vi "Draw_polygon_exercise_ms.vi"() -> ()   [LabVIEW 2016]
uses:
  Classes/Controller/Motion/A3200 Folder/A3200.lvclass
panel:
  out "XYZTheta Out 2":dbl[](array[numeric])
  out "XYZTheta Out":dbl[](array[numeric])
  in  "Speed":dbl=20.0
  out "subarray":dbl[](array[numeric])
  in  "O_y":dbl=500.0
  in  "O_x":dbl=500.0
  out "Array 2":dbl[][](array[numeric])
  out "Array":dbl[](array[numeric])
  in  "initial_angle":dbl
  out "R":dbl
  in  "r":dbl=100.0
  out "polygon_angle":dbl
  in  "P_num":i32=6
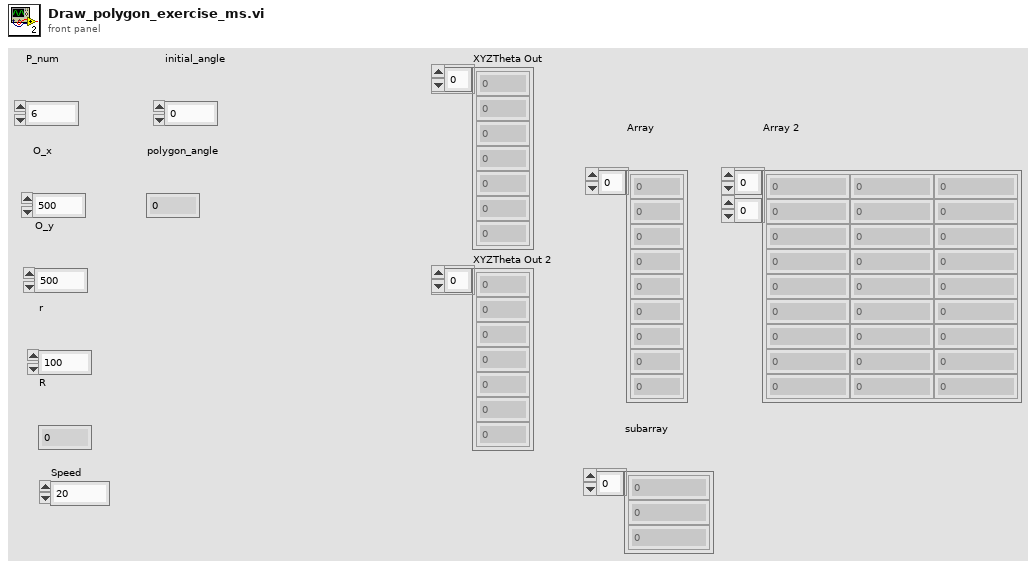
[diagram p1: front panel]
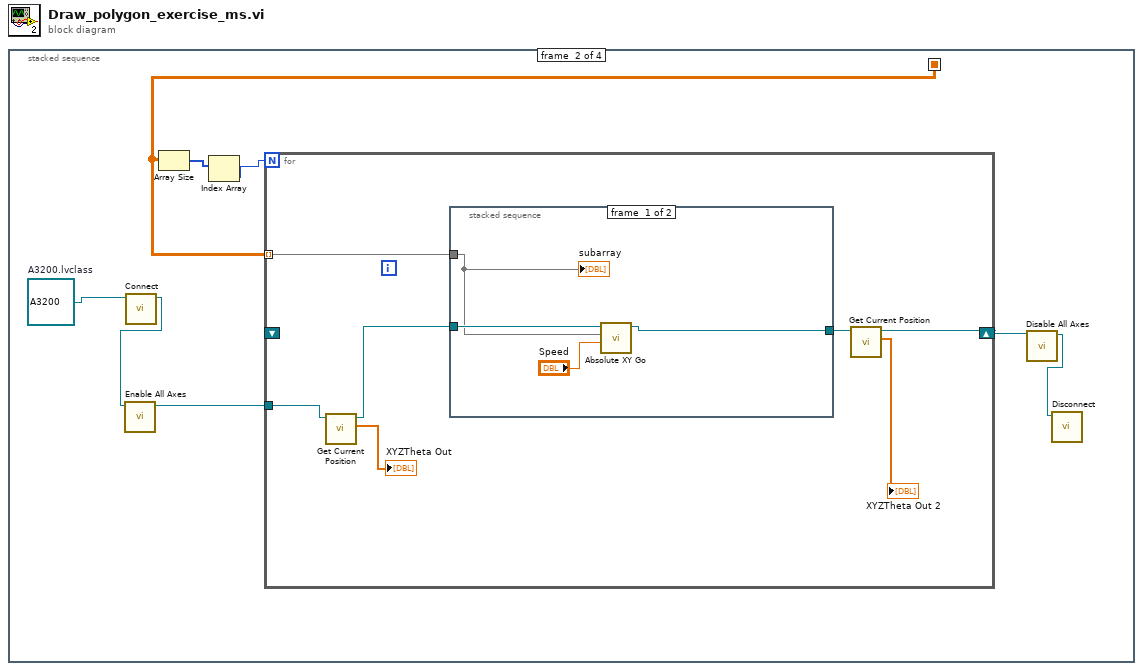
[diagram p0: block diagram]
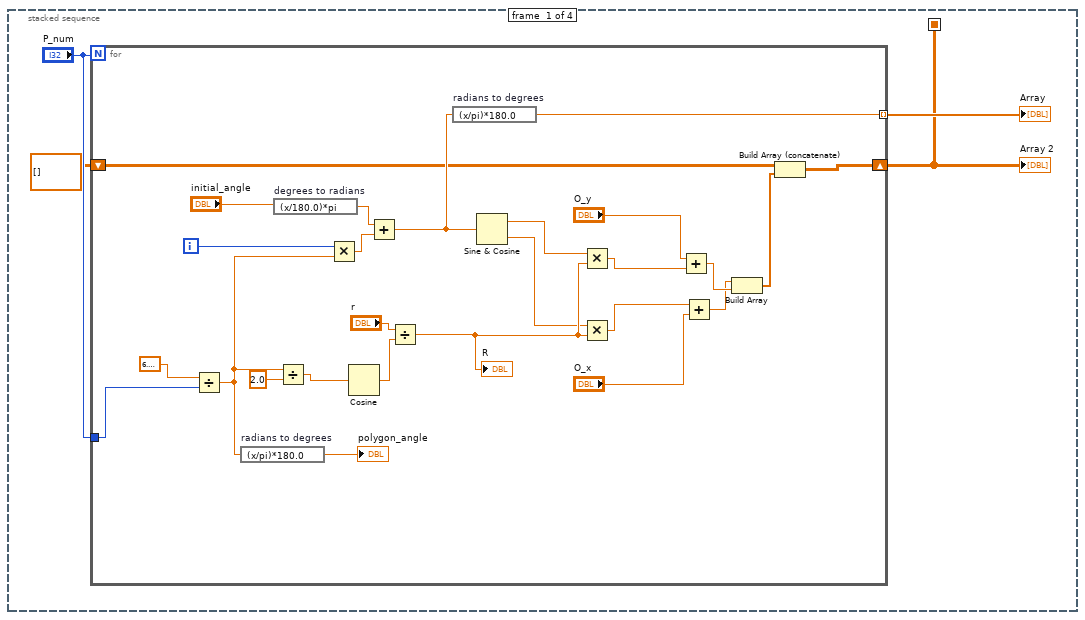
[diagram p2: hidden frame]
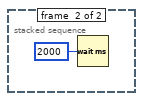
[diagram p3: hidden frame]
diagram:
  n1 = stacked-sequence {
    seq-local: [w1 _ _ _] -> [_ w36 _ _]
    frame #0 {
      n2 = for {
        N: "P_num" -> [_]
        tunnel: "P_num" -> [w27]
        tunnel: [w14] -> w3 mode=indexing
        shift-right: [w12] -> w1
        shift-left: dbl[][] [] -> [w11]
        i -> [w25]
        n3 = Divide(x=6.283185307179586, y=w27) -> (x/y=w20:dbl)
        n4 = expression code="(x/pi)*180.0" "radians to degrees"(w20) -> (→"polygon_angle":dbl)
        n5 = expression code="(x/180.0)*pi" "degrees to radians"("initial_angle") -> (w22:dbl)
        n6 = Divide(x=w20, y=2.0) -> (x/y=w18:dbl)
        n7 = Multiply(x=w25, y=w20) -> (x*y=w24:dbl)
        n8 = Cosine(x=w18) -> (cos(x)=w29:dbl)
        n9 = Add(x=w22, y=w24) -> (x+y=w15:dbl)
        n10 = Divide(x="r", y=w29) -> (x/y=w21:dbl)
        "R" <- w21
        n11 = expression code="(x/pi)*180.0" "radians to degrees"(w15) -> (w14:dbl)
        n12 = Sine & Cosine(0:w15) -> (1:w16:dbl, 2:w17:dbl)
        n13 = Multiply(x=w16, y=w21) -> (x*y=w9:dbl)
        n14 = Multiply(x=w17, y=w21) -> (x*y=w8:dbl)
        n15 = Add(x="O_y", y=w9) -> (x+y=w6:dbl)
        n16 = Add(x=w8, y="O_x") -> (x+y=w5:dbl)
        n17 = Build Array(w5, w6) -> (w13:dbl[])
        n18 = Build Array (concatenate)(w11, w13) -> (w12:dbl[][])
      }
      "Array" <- w3
      "Array 2" <- w1
    }
    frame #1 {
      w35 = refnum<class "A3200.lvclass"> refnum  # A3200.lvclass
      n19 = call-dynamic "Connect.vi"("Gantry in"=w35) -> ("Gantry out"=w34:refnum<class "A3200.lvclass">)  [unwired: 9 in, 1 out]
      n20 = call-dynamic "Enable All Axes.vi"("A3200 in"=w34) -> ("A3200 out"=w33:refnum<class "A3200.lvclass">)  [unwired: 9 in, 1 out]
      n21 = Array Size(array=w36) -> (size(s)=w38:i32[])
      n22 = Index Array(array=w38) -> (element=w37:i32)  [unwired: 1 in]
      n23 = for {
        N: w37 -> [_]
        tunnel: w36 -> [w45] mode=indexing
        tunnel: w33 -> [w44]
        shift-right: [w40] -> w31
        shift-left: _ -> [_]
        n24 = call-dynamic "Get Current Position.vi"("Gantry in"=w44) -> ("XYZTheta Out"=→"XYZTheta Out":dbl[], "Gantry out"=w43:refnum<class "A3200.lvclass">)  [unwired: 8 in, 1 out]
        n25 = stacked-sequence {
          tunnel: w45 -> [w46 _]
          tunnel: w43 -> [w49 _]
          tunnel: [w47 _] -> w41
          frame #0 {
            n26 = call-dynamic "Absolute XY Go.vi"("Speed"="Speed", "XY"=w46, "Gantry in"=w49) -> ("Gantry out"=w47:refnum<class "A3200.lvclass">)  [unwired: 7 in, 1 out]
            "subarray" <- w46
          }
          frame #1 {
            n27 = Wait (ms)(milliseconds to wait=u32 2000) -> ()  [unwired: 1 out]
          }
        }
        n28 = call-dynamic "Get Current Position.vi"("Gantry in"=w41) -> ("XYZTheta Out"=→"XYZTheta Out 2":dbl[], "Gantry out"=w40:refnum<class "A3200.lvclass">)  [unwired: 8 in, 1 out]
      }
      n29 = call-dynamic "Disable All Axes.vi"("Gantry in"=w31) -> ("Gantry out"=w32:refnum<class "A3200.lvclass">)  [unwired: 9 in, 1 out]
      n30 = call-dynamic "Disconnect.vi"("Gantry in"=w32) -> ()  [unwired: 9 in, 1 out]
    }
    frame #2 {
    }
    frame #3 {
    }
  }
